vi "Write r.vi"(8 "error in (no error)":errorcluster, 10 "r":dbl, 11 "Dot in":refnum<class "Dot.lvclass">) -> (0 "error out":errorcluster, 3 "Dot out":refnum<class "Dot.lvclass">)   [LabVIEW 2019, in "Dot.lvclass"]
uses:
  Dot.lvclass
  Dot.lvclass/Dot.ctl
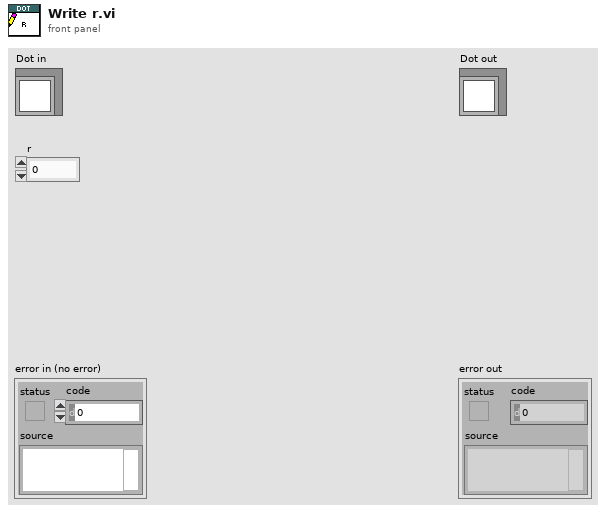
[diagram p1: front panel]
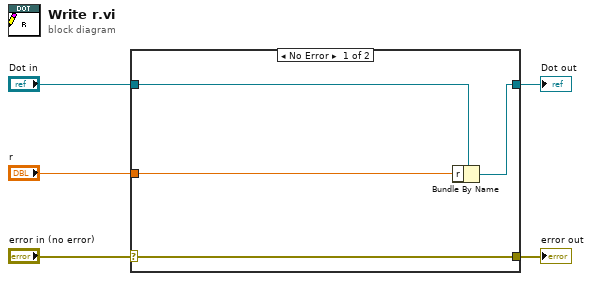
[diagram p0: block diagram]
diagram:
  n1 = case shown="No Error" "error in (no error)" {
    selector: "error in (no error)" -> [w9 w10]
    tunnel: [w9 w10] -> w4
    tunnel: [w7 w11] -> w2
    tunnel: "Dot in" -> [w8 w11]
    tunnel: "r" -> [w6 _]
    frame No Error {
      n2 = Bundle By Name(cluster=w8, "r"=w6) -> (w7:refnum<class "Dot.lvclass">)
    }
    frame Error {
    }
  }
  "error out" <- w4
  "Dot out" <- w2
